vi "Setup Result Cache.vi"(4 "Operation":enum16{"Read", "Write"}(ring), 5 "error in (no error)":errorcluster, 8 "Result":T1(ring)) -> (0 "error out":errorcluster, 3 "Result Out":T1(ring))   [LabVIEW 2020, in "StdOut Operations.lvlib"]
uses:
  StdOut Operations.lvlib
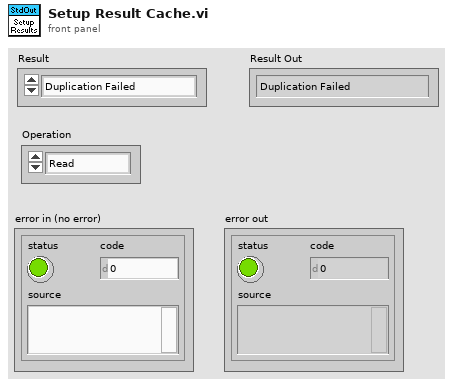
[diagram p1: front panel]
types:
  T1 = enum16{"Duplication Failed", "Duplication Succeeded"}
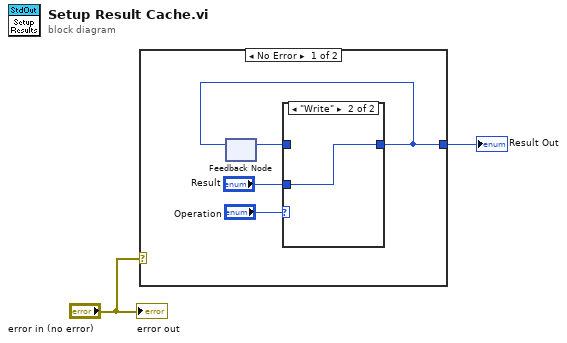
[diagram p0: block diagram]
diagram:
  n1 = case shown="No Error" "error in (no error)" {
    tunnel: [w4 _] -> w2
    frame No Error {
      n2 = feedback #1() -> (w5:T1)  [unwired: 1 in]
      n3 = case shown="\"Write\"" "Operation" {
        tunnel: w5 -> [w7 _]
        tunnel: [w7 w8] -> w4
        tunnel: "Result" -> [_ w8]
        frame "Read" {
        }
        frame "Write" {
        }
      }
      n4 = feedback-in #1(w4) -> ()
    }
    frame Error {
    }
  }
  "Result Out" <- w2
  "error out" <- "error in (no error)"
